vi "TL Motor test.vi"() -> ()   [LabVIEW 2020]
doc: "Shows how to perform a relative motor move."
panel:
  in  "MG17Motor":refnum<k7>(container)
  in  "Stop":bool
  in  "Set Rel Move Size":bool
  in  "Rel Move Size":dbl=1.0 min=-10.0 max=10.0 format="%.2f"
  in  "Move Relative":bool
  in  "Home":bool
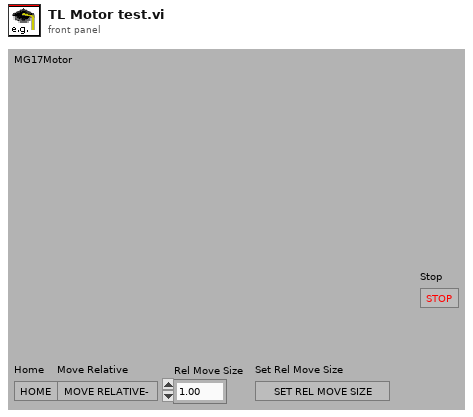
[diagram p1: front panel]
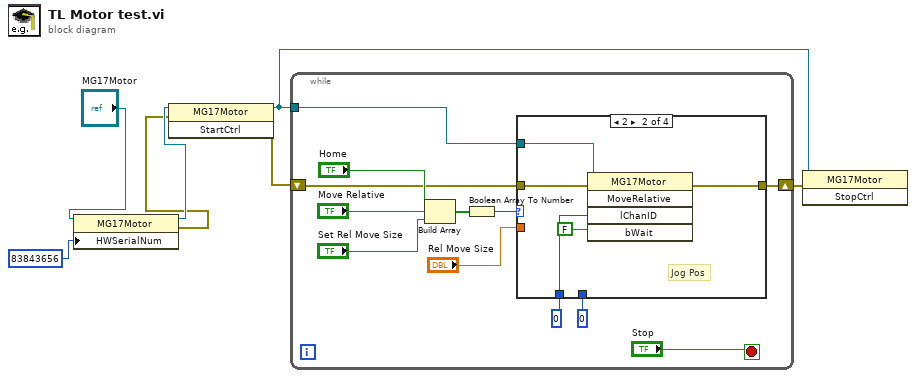
[diagram p0: block diagram]
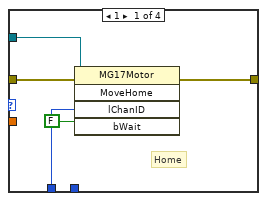
[diagram p2: hidden frame]
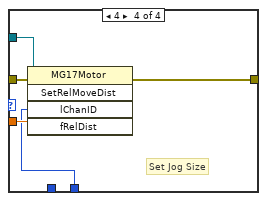
[diagram p4: hidden frame]
diagram:
  n1 = property class="MG17Motor"(reference="MG17Motor", "HWSerialNum"=83843656) -> (reference out=w2:refnum<k7>, error out=w1:errorcluster)  [unwired: 1 in]
  n2 = invoke class="MG17Motor" method="StartCtrl"(reference=w2, error in=w1) -> (reference out=w7:refnum<k7>, error out=w6:errorcluster)  [unwired: 1 in, 1 out]
  n3 = while {
    shift-left: w6 -> [w12]
    shift-right: [w13] -> w5
    tunnel: w7 -> [w17]
    stop <- "Stop" stop-if-true
    n4 = Build Array("Home", "Move Relative", "Set Rel Move Size") -> (w9:bool[])
    n5 = Boolean Array To Number(Boolean array=w9) -> (number=w10:u32)
    n6 = case shown="2" w10 {
      tunnel: w17 -> [w24 w29 _ w35]
      tunnel: 0 ("lChanID") -> [w23 w28 _ _]
      tunnel: "Rel Move Size" -> [_ _ _ w34]
      tunnel: [w22 w27 w30 w32] -> w13
      tunnel: w12 -> [w21 w25 w30 w31]
      tunnel: 0 ("lChanID") -> [_ _ _ w33]
      frame 1 {
        # "Home"
        n7 = invoke class="MG17Motor" method="MoveHome"(reference=w24, error in=w21, "lChanID"=w23, "bWait"=FALSE) -> (error out=w22:errorcluster)  [unwired: 1 in, 4 out]
      }
      frame 2 {
        # "Jog Pos"
        n8 = invoke class="MG17Motor" method="MoveRelative"(reference=w29, error in=w25, "lChanID"=w28, "bWait"=FALSE) -> (error out=w27:errorcluster)  [unwired: 1 in, 4 out]
      }
      frame Default {
      }
      frame 4 {
        # "Set Jog Size"
        n9 = invoke class="MG17Motor" method="SetRelMoveDist"(reference=w35, error in=w31, "lChanID"=w33, "fRelDist"=w34) -> (error out=w32:errorcluster)  [unwired: 1 in, 4 out]
      }
    }
  }
  n10 = invoke class="MG17Motor" method="StopCtrl"(reference=w7, error in=w5) -> ()  [unwired: 1 in, 3 out]
